vi "myRIO_BRig_FPGA_CueLed__v2.vi"(1 "I_peak":bool, 2 "count":u32, 4 "laser_Npeak":u32=100, 5 "laser_Nvalley":u32=100, 6 "I_CueLed_Event":bool) -> (15 "output_I_peak":bool, 16 "output_count":u32, 18 "output_led":bool)   [LabVIEW 2014]
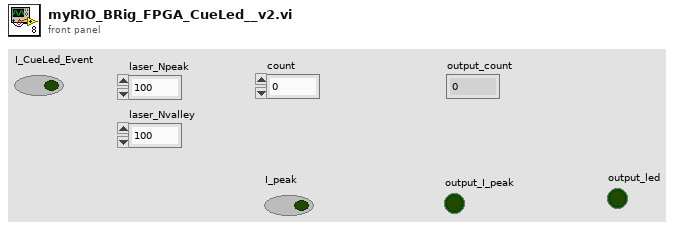
[diagram p1: front panel]
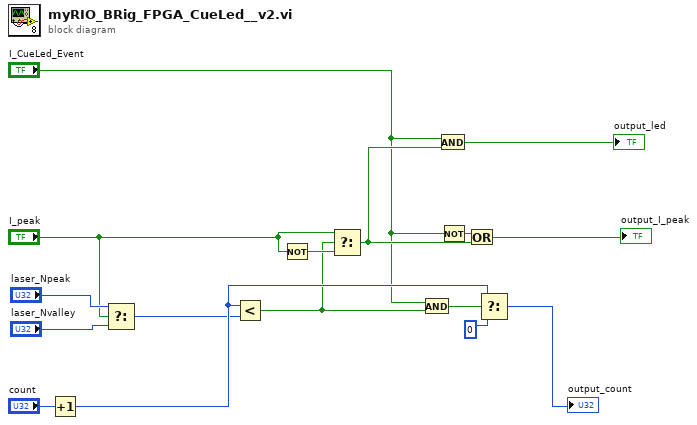
[diagram p0: block diagram]
diagram:
  n1 = Increment(x="count") -> (x+1=w13:u32)
  n2 = Select(t="laser_Npeak", s="I_peak", f="laser_Nvalley") -> (s? t:f=w6:u32)
  n3 = Less?(x=w13, y=w6) -> (x < y?=w2:bool)
  n4 = Not(x="I_peak") -> (.not. x?=w5:bool)
  n5 = Select(t="I_peak", s=w2, f=w5) -> (s? t:f=w8:bool)
  n6 = And(x="I_CueLed_Event", y=w2) -> (x .and. y?=w3:bool)
  n7 = And(x="I_CueLed_Event", y=w8) -> (x .and. y?=→"output_led":bool)
  n8 = Not(x="I_CueLed_Event") -> (.not. x?=w7:bool)
  n9 = Or(x=w7, y=w8) -> (x .or. y?=→"output_I_peak":bool)
  n10 = Select(t=w13, s=w3, f=u32 0) -> (s? t:f=→"output_count":u32)
